vi "PhotonCamera_TakeOutputSnapshot.vi"(11 "CameraName":string) -> ()   [LabVIEW 2019, in "PhotonVisionLib.lvlib"]
doc: "Request the camera to save a new image file from the output stream with overlays. Images take up space in the filesystem of the PhotonCamera. Calling it frequently will fill up disk space and eventually cause the system to stop working. Clear out images in /opt/photonvision/photonvision_config/imgSaves frequently to prevent issues.\n\nInputs:\n - CameraName -- The nickname of the camera (found in the PhotonVision UI).\n\nOutputs:\n - >none<"
uses:
  PhotonVisionLib.lvlib
  <vilib>/Rock Robotics/Network Tables/NT Write Boolean.vi
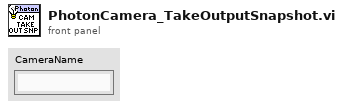
[diagram p1: front panel]
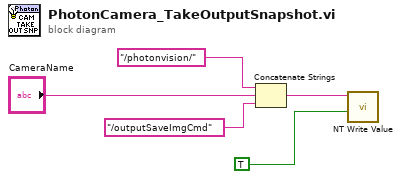
[diagram p0: block diagram]
diagram:
  n1 = Concatenate Strings("/photonvision/", "CameraName", "/outputSaveImgCmd") -> (w2:string)
  n2 = call-poly <vilib>:"NT Write Value.vi"("Boolean"=TRUE, "Name"=w2) -> ()  [unwired: 9 in, 1 out]
